vi "Delete_PKYK.vi"(8 "error in (no error)":errorcluster, 10 "PokaYoke In":T1 {"MachineCode" items=["MCIG", "MCPC", "MCSA", "MCCA", "MCAC", "MCLA", "MCCM", "MCSC", "MCPA", "MCLP", "MCHP", "MCBC", "MCFA", "MCSR", "MCFV"]; "ExpiryDate" format="%<%I:%M:%S%3u %p\n%d-%m-%Y>T"; "EntDt" format="%<%I:%M:%S%3u %p\n%d-%m-%Y>T"; "UpdDt" format="%<%I:%M:%S%3u %p\n%d-%m-%Y>T"}, 11 "Refnum in":T6) -> (0 "error out":errorcluster, 3 "Refnum out":T6)   [LabVIEW 2020]
uses:
  <vilib>/addons/database/Connection.llb/Conn ObjectReference.ctl
  Controls/Line_PKYK.ctl
  Controls/PARA_CONTROL_STR.ctl
  Controls/PKYK_MCODE.ctl
  Controls/PKYK_DATE.ctl
  Controls/PKYK_Result.ctl
  <vilib>/addons/database/NI_Database_API.lvlib
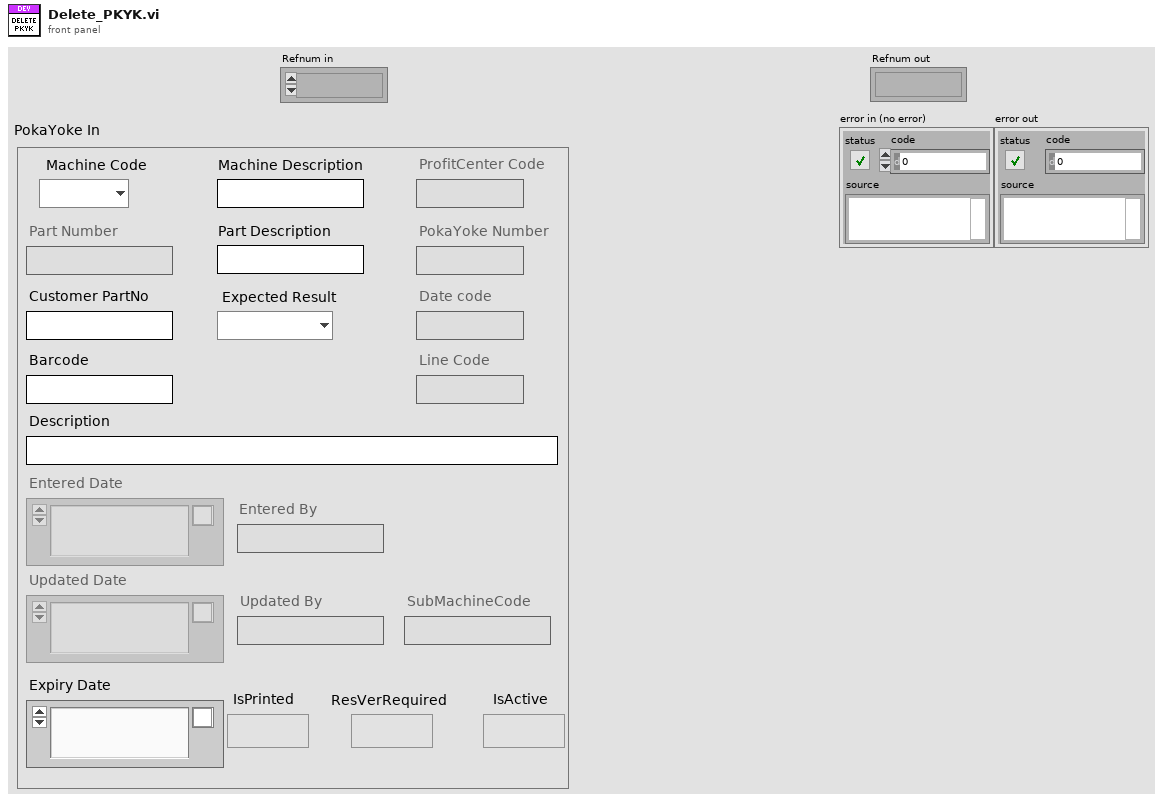
[diagram p1: front panel]
types:
  T1 = typedef "Line_PKYK.ctl" = cluster{"ProfitCenterCode":string, "LineCode":string, "Datecode":string, "PartNumber":T2, "PartDescription":T2, "CustPartNo":T2, "MachineCode":T3, "MachineDescription":T2, "PokaYokeNumber":string, "Description":string, "ExpiryDate":T4, "Barcode":T2, "IsPrinted":bool, "IsActive":bool, "EntBy":T2, "EntDt":T4, "UpdBy":T2, "UpdDt":T4, "ExpResult":T5, "ResVerRequired":bool, "SubMachineCode":T2}
  T2 = typedef "PARA_CONTROL_STR.ctl" = string
  T3 = typedef "PKYK_MCODE.ctl" = u16
  T4 = typedef "PKYK_DATE.ctl" = timestamp
  T5 = typedef "PKYK_Result.ctl" = enum16{"FAIL", "PASS"}
  T6 = typedef "NI_Database_API.lvlib/Conn ObjectReference.ctl" = refnum<k1>
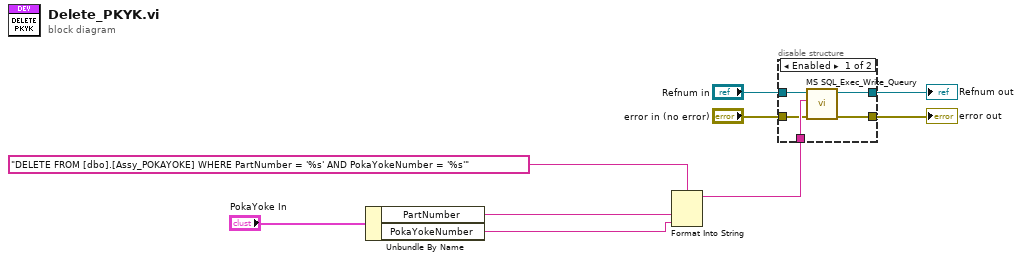
[diagram p0: block diagram]
diagram:
  n1 = Unbundle By Name("PokaYoke In") -> ("PartNumber"=w3:T2, "PokaYokeNumber"=w2:string)
  n2 = Format Into String(format string="DELETE FROM [dbo].[Assy_POKAYOKE] WHERE PartNumber = '%s' AND PokaYokeNumber = '%s'", w3, w2) -> (resulting string=w8:string)  [unwired: 2 in, 1 out]
  n3 = disable-structure shown="Enabled" {
    disable-tunnel: w8 -> [w14 _]
    disable-tunnel: "Refnum in" -> [w13 w15]
    disable-tunnel: [w12 w15] -> w6
    disable-tunnel: "error in (no error)" -> [w11 _]
    disable-tunnel: [w10 _] -> w4
    frame Enabled {
      n4 = call "MS SQL_Exec_Write_Queury.vi"("error in (no error)"=w11, "Query"=w14, "Refnum in"=w13) -> ("error out"=w10:errorcluster, "Refnum out"=w12:T6)  [unwired: 7 in]
    }
    frame Disabled {
    }
  }
  "Refnum out" <- w6
  "error out" <- w4
